vi "CRYMR_Move.vi"(1 "Input":cluster{dbl, dbl}[](array[cluster]) {"?" format="%.2f"; "?" format="%.2f"}, 2 "Offsets":cluster{"X Offset":dbl, "Y Offset":dbl} {"Y Offset" format="%.2f"; "X Offset" format="%.2f"}) -> (0 "Output":cluster{dbl, dbl}[](array[cluster]) {"?" format="%.2f"; "?" format="%.2f"})   [LabVIEW 2013]
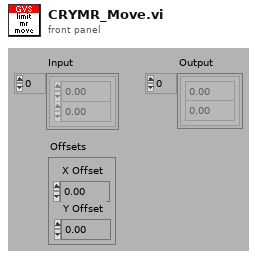
[diagram p1: front panel]
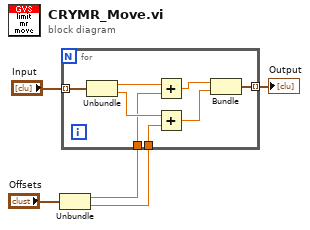
[diagram p0: block diagram]
diagram:
  n1 = Unbundle("Offsets") -> ("X Offset"=w2:dbl, "Y Offset"=w1:dbl)
  n2 = for {
    tunnel: "Input" -> [w13] mode=indexing
    tunnel: [w11] -> w4 mode=indexing
    tunnel: w2 -> [w7]
    tunnel: w1 -> [w6]
    n3 = Unbundle(w13) -> (w9:dbl, w8:dbl)
    n4 = Add(x=w9, y=w7) -> (x+y=w12:dbl)
    n5 = Add(x=w8, y=w6) -> (x+y=w10:dbl)
    n6 = Bundle(w12, w10) -> (w11:cluster{dbl, dbl})  [unwired: 1 out]
  }
  "Output" <- w4
